vi "LabVIEW Basics.vi"() -> ()   [LabVIEW 2019]
panel:
  out "x+y":dbl
  out "B":dbl
  out "A":dbl
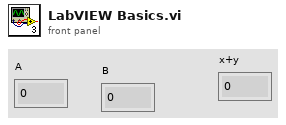
[diagram p1: front panel]
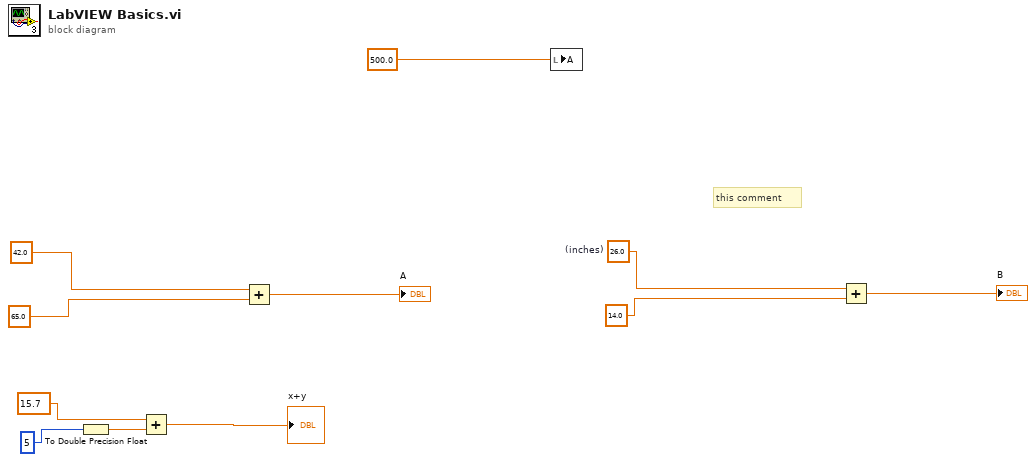
[diagram p0: block diagram]
diagram:
  w7 = 26.0  # (inches)
  # "this comment"
  n1 = To Double Precision Float(number=5) -> (double precision float=w1:dbl)
  n2 = Add(x=15.7, y=w1) -> (x+y=→"x+y":dbl)
  n3 = Add(x=42.0, y=65.0) -> (x+y=→"A":dbl)
  n4 = local write "A"(500.0 ("A")) -> ()
  n5 = Add(x=w7, y=14.0) -> (x+y=→"B":dbl)
